vi "2_4_Linear system property.vi"() -> ()   [LabVIEW 2009]
panel:
  out "System":T1(ring)
  out "System":T1(ring)
  in  "System":T1(ring)
  in  "stop":bool
  in  "b":dbl=3.0
  in  "a":dbl=2.0
  in  "Signal 2: x2[n]":dbl[](array[numeric])=[1.0, 1.0, 1.0, 1.0, 1.0]
  in  "Signal 1: x1[n]":dbl[](array[numeric])=[2.0, 1.0, 2.0, 3.0, 1.0]
  out "Output y2[n]":dbl[](graph)=[7.0, 12.0, 19.0, 28.0, 33.0]
  out "Output y1[n]":dbl[](graph)=[7.0, 12.0, 19.0, 28.0, 33.0]
  # "Linear Systems Property:"
  # "Program Developed by Indranil Sinharoy"
  # "a.x1[n]"
  # "y2[n]"
  # "b.x2[n]"
  # "+"
  # "a.x1[n]"
  # "y1[n]"
  # "b.x2[n]"
  # "+"
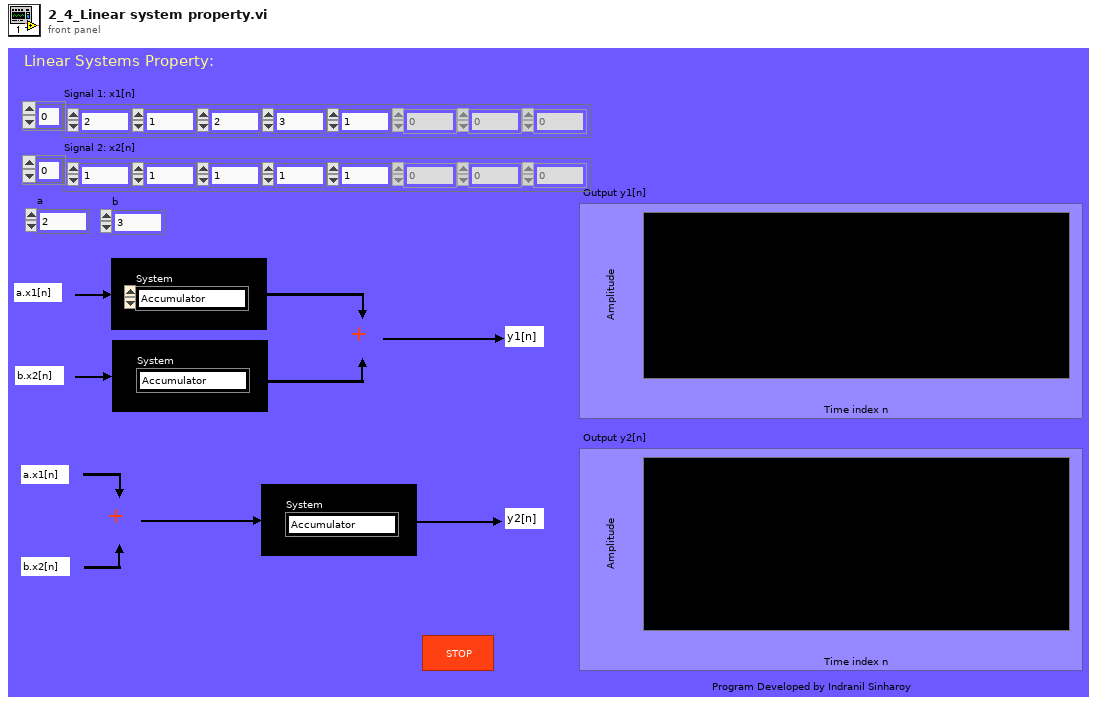
[diagram p1: front panel]
types:
  T1 = enum16{"Accumulator", "Moving Avg", "Causal Delay", "Square"}
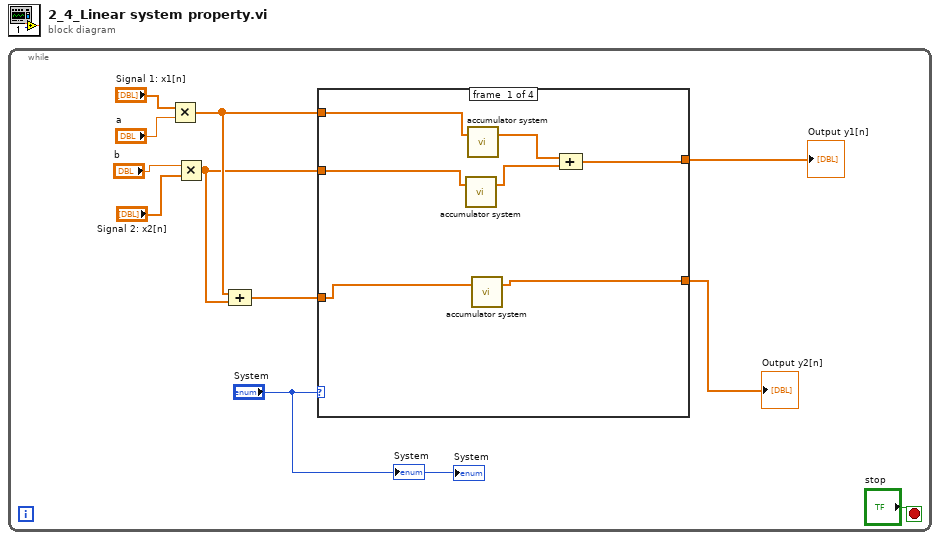
[diagram p0: block diagram]
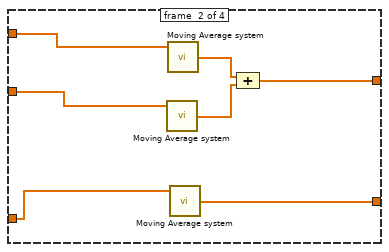
[diagram p2: hidden frame]
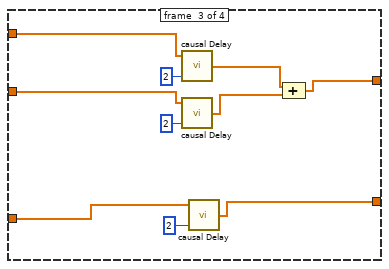
[diagram p3: hidden frame]
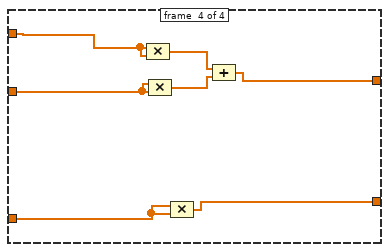
[diagram p4: hidden frame]
diagram:
  n1 = while {
    stop <- "stop" stop-if-true
    n2 = Multiply(x="Signal 1: x1[n]", y="a") -> (x*y=w6:dbl[])
    n3 = Multiply(x="b", y="Signal 2: x2[n]") -> (x*y=w5:dbl[])
    n4 = Compound Arithmetic op=ADD(w6, w5) -> (w11:dbl[])
    n5 = case shown="\"Square\"" "System" {
      tunnel: w11 -> [w13 w23 w27 w37]
      tunnel: w6 -> [w17 w25 w34 w41]
      tunnel: w5 -> [w18 w24 w32 w42]
      tunnel: [w14 w20 w29 w38] -> w2
      tunnel: [w12 w19 w26 w36] -> w1
      frame #0 {
        n6 = call "accumulator system.vi"("Sequence x[n]"=w18) -> ("Accumulated sequence A[n] = Sum(k: k ( -infinity to n) x[k]"=w15:dbl[])  [unwired: 2 out]
        n7 = call "accumulator system.vi"("Sequence x[n]"=w17) -> ("Accumulated sequence A[n] = Sum(k: k ( -infinity to n) x[k]"=w16:dbl[])  [unwired: 2 out]
        n8 = call "accumulator system.vi"("Sequence x[n]"=w13) -> ("Accumulated sequence A[n] = Sum(k: k ( -infinity to n) x[k]"=w12:dbl[])  [unwired: 2 out]
        n9 = Compound Arithmetic op=ADD(w16, w15) -> (w14:dbl[])
      }
      frame #1 {
        n10 = call "Moving Average system.vi"("Input Signal"=w24) -> ("Moving Average Output"=w21:dbl[])  [unwired: 2 in]
        n11 = call "Moving Average system.vi"("Input Signal"=w25) -> ("Moving Average Output"=w22:dbl[])  [unwired: 2 in]
        n12 = call "Moving Average system.vi"("Input Signal"=w23) -> ("Moving Average Output"=w19:dbl[])  [unwired: 2 in]
        n13 = Compound Arithmetic op=ADD(w22, w21) -> (w20:dbl[])
      }
      frame #2 {
        n14 = call "causal Delay.vi"("DELAY"=2, "X"=w34) -> ("Delayed sequence"=w31:dbl[])
        n15 = call "causal Delay.vi"("DELAY"=2, "X"=w32) -> ("Delayed sequence"=w30:dbl[])
        n16 = call "causal Delay.vi"("DELAY"=2, "X"=w27) -> ("Delayed sequence"=w26:dbl[])
        n17 = Compound Arithmetic op=ADD(w31, w30) -> (w29:dbl[])
      }
      frame #3 {
        n18 = Compound Arithmetic op=MULTIPLY(w41, w41) -> (w40:dbl[])
        n19 = Compound Arithmetic op=MULTIPLY(w42, w42) -> (w39:dbl[])
        n20 = Compound Arithmetic op=MULTIPLY(w37, w37) -> (w36:dbl[])
        n21 = Compound Arithmetic op=ADD(w40, w39) -> (w38:dbl[])
      }
    }
    "Output y1[n]" <- w2
    "Output y2[n]" <- w1
    "System" <- "System"
    "System" <- "System"
  }
